vi "Database.Main.vi"() -> ()   [LabVIEW 2016]
uses:
  Database.Main.Data.ctl
  Database.Main.Data.Status.ctl
  Database.Main.Data.Sets.ctl
  Database.Main.Data.Results.ctl
  Sequence/Sequence.Step.Status.ctl
  ProdaNG/Controls/ProdaNG.Identification.ctl
  ProdaNG/Controls/ProdaNG.ProcessResult.ctl
  ProdaNG/Controls/ProdaNG.ProcessStepResult.ctl
  ProdaNG/Controls/ProdaNG.TestStepResult.ctl
  ProdaNG/Controls/ProdaNG.TestValueResult.ctl
  Database.Main.Data.Variant.ctl
  ProdaNG/Controls/ProdaNG.ProcessStepParam.ctl
  ProdaNG/Controls/ProdaNG.TestStep.ctl
  ProdaNG/Controls/ProdaNG.TestStepParam.ctl
  ProdaNG/Controls/ProdaNG.TestValue.ctl
  Database.Main.Action.ctl
  tools/CitTemplate/citTemplate.errData.ctl
  tools/EventLog/EventLog.EventSource.ctl
  Database.Global.vi
panel:
  out "LastFile":string
  out "error.action":string
  out "error":errorcluster
  out "_loop":i32(ring)=4
  out "action":T1=enum."--- DB ---"
  out "Data":T2 {"Variant"."TS"."TV"."minimum" format="%#.3f"; "Variant"."TS"."TV"."maximum" format="%#.3f"; "Variant"."TS"."TP"."value" format="%#.3f"}
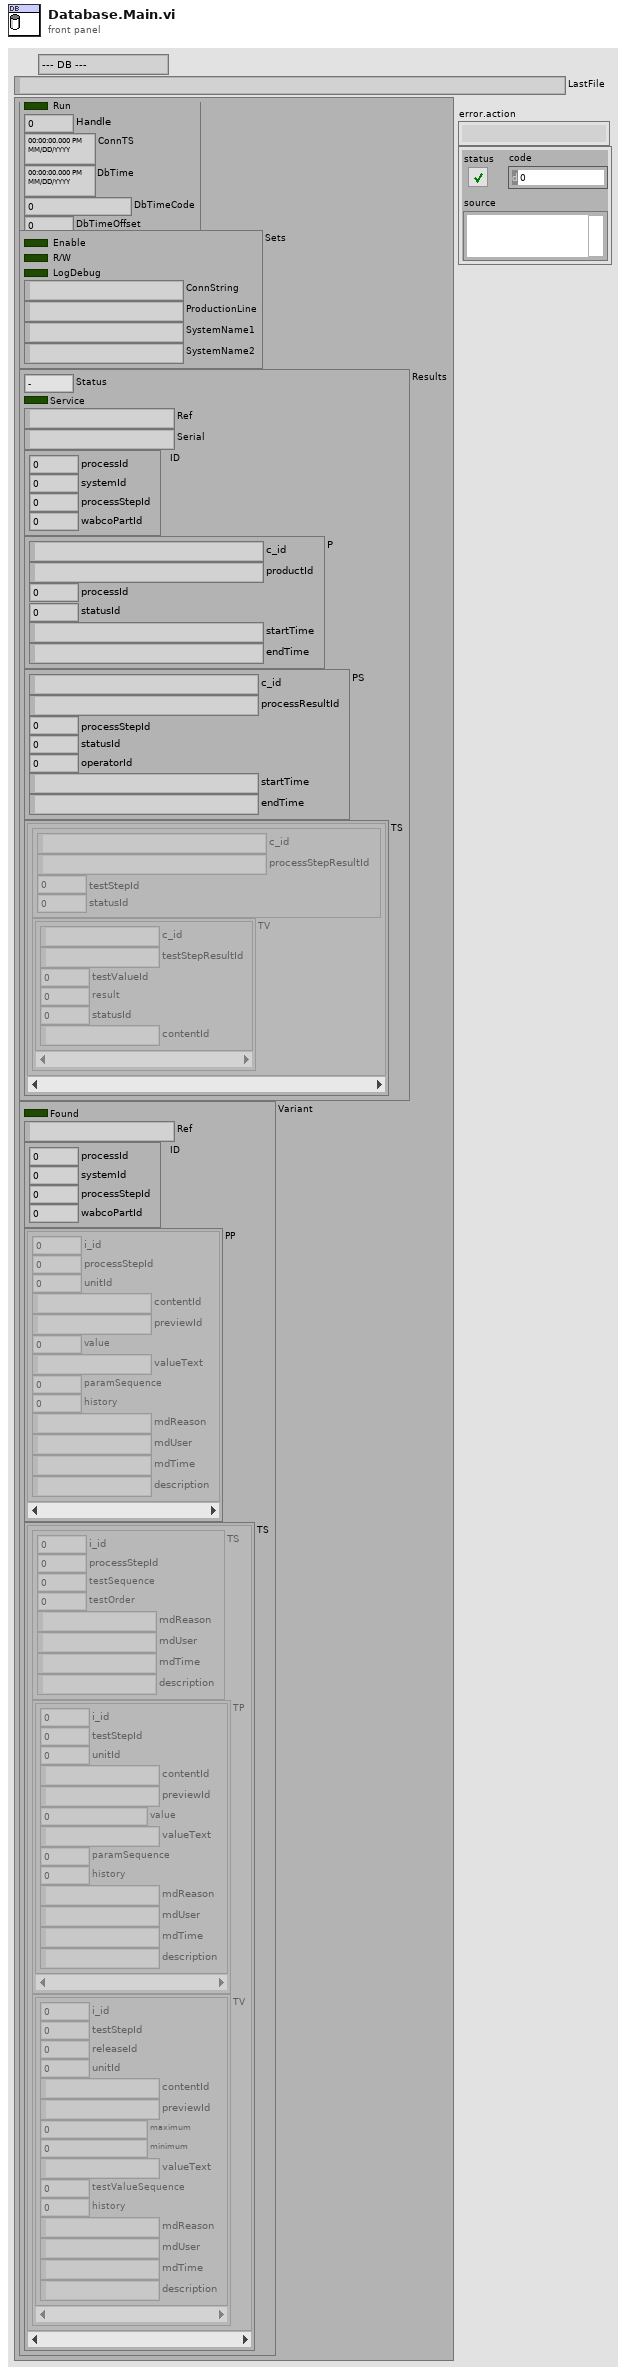
[diagram p1: front panel]
types:
  T1 = typedef "Database.Main.Action.ctl" = enum32{"idle", "constructor", "destructor", "--- DB ---", "Init", "Setup", "Select.Variant", "File.Export"}
  T2 = typedef "Database.Main.Data.ctl" = cluster{"Status":T3, "Sets":T4, "Results":T5, "Variant":T12}
  T3 = typedef "Database.Main.Data.Status.ctl" = cluster{"Run":bool, "Handle":i32, "ConnTS":timestamp, "DbTime":timestamp, "DbTimeCode":dbl, "DbTimeOffset":dbl}
  T4 = typedef "Database.Main.Data.Sets.ctl" = cluster{"Enable":bool, "R/W":bool, "LogDebug":bool, "ConnString":string, "ProductionLine":string, "SystemName1":string, "SystemName2":string}
  T5 = typedef "Database.Main.Data.Results.ctl" = cluster{"Status":T6, "Service":bool, "Ref":string, "Serial":string, "ID":T7, "P":T8, "PS":T9, "TS":cluster{"TS":T10, "TV":T11[]}[]}
  T6 = typedef "Sequence.Step.Status.ctl" = enum16{"-", "Pending", "Running", "Skipped", "Passed", "Failed", "Done", "Error", "Aborted", "Stopped"}
  T7 = typedef "ProdaNG.Identification.ctl" = cluster{"processId":i32, "systemId":i32, "processStepId":i32, "wabcoPartId":i32}
  T8 = typedef "ProdaNG.ProcessResult.ctl" = cluster{"c_id":string, "productId":string, "processId":i32, "statusId":i32, "startTime":string, "endTime":string}
  T9 = typedef "ProdaNG.ProcessStepResult.ctl" = cluster{"c_id":string, "processResultId":string, "processStepId":i32, "statusId":i32, "operatorId":i32, "startTime":string, "endTime":string}
  T10 = typedef "ProdaNG.TestStepResult.ctl" = cluster{"c_id":string, "processStepResultId":string, "testStepId":i32, "statusId":i32}
  T11 = typedef "ProdaNG.TestValueResult.ctl" = cluster{"c_id":string, "testStepResultId":string, "testValueId":i32, "result":dbl, "statusId":i32, "contentId":string}
  T12 = typedef "Database.Main.Data.Variant.ctl" = cluster{"Found":bool, "Ref":string, "ID":T7, "PP":T13[], "TS":cluster{"TS":T14, "TP":T15[], "TV":T16[]}[]}
  T13 = typedef "ProdaNG.ProcessStepParam.ctl" = cluster{"i_id":i32, "processStepId":i32, "unitId":i32, "contentId":string, "previewId":string, "value":dbl, "valueText":string, "paramSequence":i32, "history":i32, "mdReason":string, "mdUser":string, "mdTime":string, "description":string}
  T14 = typedef "ProdaNG.TestStep.ctl" = cluster{"i_id":i32, "processStepId":i32, "testSequence":i32, "testOrder":i32, "mdReason":string, "mdUser":string, "mdTime":string, "description":string}
  T15 = typedef "ProdaNG.TestStepParam.ctl" = cluster{"i_id":i32, "testStepId":i32, "unitId":i32, "contentId":string, "previewId":string, "value":dbl, "valueText":string, "paramSequence":i32, "history":i32, "mdReason":string, "mdUser":string, "mdTime":string, "description":string}
  T16 = typedef "ProdaNG.TestValue.ctl" = cluster{"i_id":i32, "testStepId":i32, "releaseId":i32, "unitId":i32, "contentId":string, "previewId":string, "maximum":dbl, "minimum":dbl, "valueText":string, "testValueSequence":i32, "history":i32, "mdReason":string, "mdUser":string, "mdTime":string, "description":string}
  T17 = typedef "citTemplate.errData.ctl" = cluster{"ts":timestamp, "src":T18, "instance":i32, "action":string, "error":errorcluster, "unconfirmed":bool}
  T18 = typedef "EventLog.EventSource.ctl" = enum16{"All", "Gui", "Ref", "File", "Arch", "Seq", "CPX", "DB", "Laser", "Scan.P", "Scan.O"}
  T19 = typedef "citTemplate.notifierHandle.ctl" = refnum<notifier>
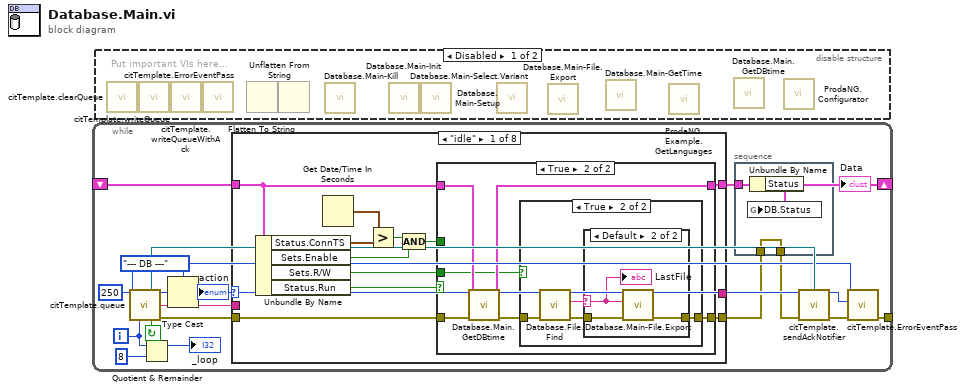
[diagram p0: block diagram]
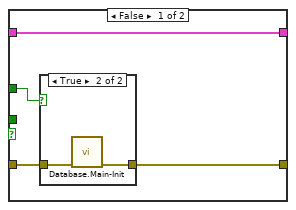
[diagram p3: hidden frame]
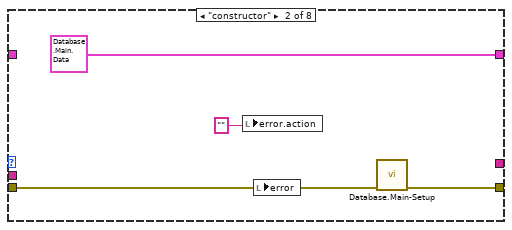
[diagram p7: hidden frame]
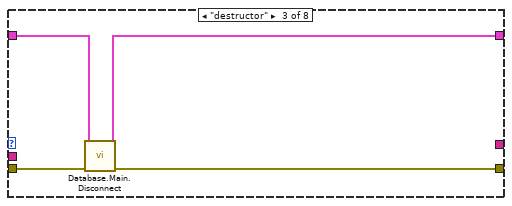
[diagram p8: hidden frame]
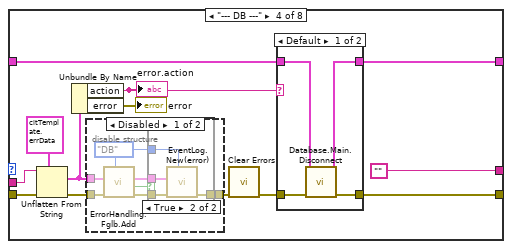
[diagram p9: hidden frame]
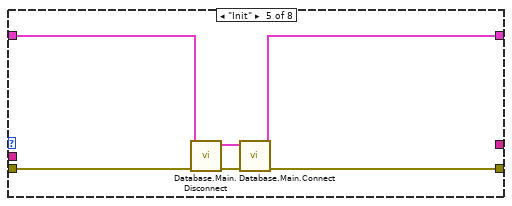
[diagram p13: hidden frame]
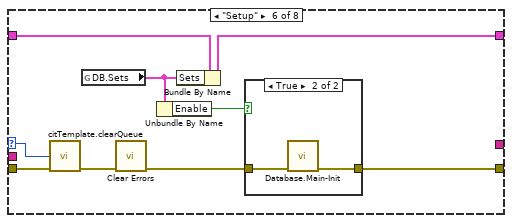
[diagram p14: hidden frame]
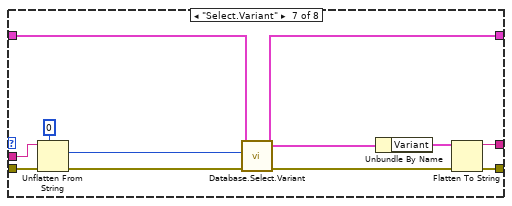
[diagram p16: hidden frame]
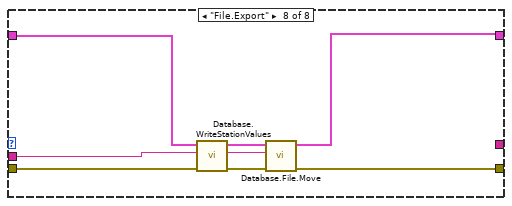
[diagram p17: hidden frame]
diagram:
  n1 = while {
    tunnel: [w11] -> _
    shift-right: [w8] -> _
    shift-left: _ -> [w1]
    i -> [w12]
    stop <- w14 continue-if-true
    w4 = Database.Main.Action."--- DB ---" ("Action")
    n2 = call "citTemplate.queue.vi"("ms timeout (250 ms)"=250, "event enum"=w4, "iteration (-1)"=w12) -> ("notifierHandle out"=w5:T19, "event out"=w17:u32, "(flatten) data out"=w16:string, "continue"=w14:bool, "error out"=w15:errorcluster)  [unwired: 2 in, 6 out]
    n3 = Quotient & Remainder(x=w12, y=8) -> (x-y*floor(x/y)=→"_loop":i32)  [unwired: 1 out]
    n4 = Type Cast(type=w4, x=w17) -> (*(type *) &x=w10:T1)
    "action" <- w10
    n5 = case shown="\"idle\"" w10 {
      selector: w10 -> [_ _ _ _ _ w106 _ _]
      tunnel: w16 -> [_ _ _ w68 _ _ w120 w124]
      tunnel: w15 -> [w29 w54 w59 w74 w94 w107 w121 w128]
      tunnel: [w26 w57 w58 w70 w98 w103 w116 w125] -> w3
      tunnel: [w24 T2 {"Status"={"Run"=FALSE, "Handle"=0, "ConnTS"=timestamp(0 s since 1904-01-01), "DbTime"=timestamp(0 s since 1904-01-01), "DbTimeCode"=0.0, "DbTimeOffset"=0.0}, "Sets"={"Enable"=FALSE, "R/W"=FALSE, "LogDebug"=FALSE, "ConnString"="", "ProductionLine"="", "SystemName1"="", "SystemName2"=""}, "Results"={"Status"=enum."-", "Service"=FALSE, "Ref"="", "Serial"="", "ID"={"processId"=0, "systemId"=0, "processStepId"=0, "wabcoPartId"=0}, "P"={"c_id"="", "productId"="", "processId"=0, "statusId"=0, "startTime"="", "endTime"=""}, "PS"={"c_id"="", "processResultId"="", "processStepId"=0, "statusId"=0, "operatorId"=0, "startTime"="", "endTime"=""}, "TS"=[]}, "Variant"={"Found"=FALSE, "Ref"="", "ID"={"processId"=0, "systemId"=0, "processStepId"=0, "wabcoPartId"=0}, "PP"=[], "TS"=[]}} ("Data") w60 w71 w97 w101 w111 w127] -> w8
      tunnel: w1 -> [w25 _ w61 w72 w93 w102 w118 w126]
      tunnel: [_ _ _ "" _ _ w115 _] -> w6
      frame "idle" {
        n6 = Unbundle By Name(w25) -> ("Status.ConnTS"=w30:timestamp, "Sets.Enable"=w22:bool, "Sets.R/W"=w21:bool, "Status.Run"=w27:bool)
        n7 = Get Date/Time In Seconds() -> (seconds since 1Jan1904=w31:timestamp)
        n8 = Greater?(x=w31, y=w30) -> (0:w28:bool)
        n9 = Compound Arithmetic op=AND(w28, w22) -> (w23:bool)
        n10 = case shown="True" w27 {
          tunnel: w29 -> [w35 w42]
          tunnel: w23 -> [w34 _]
          tunnel: [w33 w40] -> w26
          tunnel: w25 -> [w32 w44]
          tunnel: [w32 w43] -> w24
          tunnel: w21 -> [_ w39]
          frame False {
            n11 = case shown="True" w34 {
              tunnel: w35 -> [w36 w38]
              tunnel: [w36 w37] -> w33
              frame False {
              }
              frame True {
                n12 = call "Database.Main-Init.vi"("error in"=w38) -> ("error out"=w37:errorcluster)  [unwired: 10 in]
              }
            }
          }
          frame True {
            n13 = call "Database.Main.GetDBtime.vi"("error in (no error)"=w42, "Data in"=w44) -> ("error out"=w41:errorcluster, "Data out"=w43:T2)  [unwired: 8 in]
            n14 = case shown="True" w39 {
              tunnel: w41 -> [w45 w49]
              tunnel: [w45 w48] -> w40
              frame False {
              }
              frame True {
                n15 = call "Database.File.Find.vi"("error in (no error)"=w49) -> ("error out"=w47:errorcluster, "FileName"=w46:string)  [unwired: 9 in]
                n16 = case shown="Default" w46 {
                  selector: w46 -> [_ w51]
                  tunnel: w47 -> [w50 w53]
                  tunnel: [w50 w52] -> w48
                  frame "" {
                  }
                  frame Default {
                    n17 = call "Database.Main-File.Export.vi"("error in"=w53, "FileName"=w51) -> ("error out"=w52:errorcluster)  [unwired: 9 in]
                    "LastFile" <- w51
                  }
                }
              }
            }
          }
        }
      }
      frame "constructor" {
        n18 = local write "error.action"("" ("error.action")) -> ()
        n19 = local write "error"(w54) -> ()
        n20 = call "Database.Main-Setup.vi"("error in"=w54) -> ("error out"=w57:errorcluster)  [unwired: 10 in]
      }
      frame "destructor" {
        n21 = call "Database.Main.Disconnect.vi"("error in (no error)"=w59, "Data in"=w61) -> ("error out"=w58:errorcluster, "Data out"=w60:T2)  [unwired: 8 in]
      }
      frame "--- DB ---" {
        n22 = Unflatten From String(type=T17 {"ts"=timestamp(0 s since 1904-01-01), "src"=enum."All", "instance"=0, "action"="", "error"={"status"=FALSE, "code"=0, "source"=""}, "unconfirmed"=FALSE} ("ErrData"), binary string=w68, error in (no error)=w74) -> (value=w63:T17, error out=w66:errorcluster)  [unwired: 3 out]
        n23 = Unbundle By Name(w63) -> ("action"=w62:string, "error"=→"error":errorcluster)
        "error.action" <- w62
        n24 = disable-structure shown="Disabled" {
          disable-tunnel: w66 -> [w78 w86]
          disable-tunnel: [w76 w86] -> w65
          disable-tunnel: w63 -> [w75 _]
          frame Disabled {
            w77 = EventLog.EventSource."DB" ("Event source")
            n25 = call "ErrorHandling.Fglb.Add.vi"("Event source"=w77, "error in (no error)"=w78, "Error in"=w75) -> ("error out"=w80:errorcluster, "changed?"=w79:bool)  [unwired: 7 in]
            n26 = case shown="True" w79 {
              tunnel: [w81 w85] -> w76
              tunnel: w75 -> [_ w84]
              tunnel: w80 -> [w81 w83]
              tunnel: w77 -> [_ w82]
              frame False {
              }
              frame True {
                n27 = call "EventLog.New(error).vi"("Source (All)"=w82, "error in"=w83, "ErrData"=w84) -> ("error out"=w85:errorcluster)  [unwired: 8 in]
              }
            }
          }
          frame Enabled {
          }
        }
        n28 = call <vilib>:"Clear Errors.vi"("error in (no error)"=w65) -> ("error out"=w69:errorcluster)  [unwired: 5 in, 1 out]
        n29 = case shown="Default" w62 {
          tunnel: w72 -> [w90 w91]
          tunnel: [w89 w91] -> w71
          tunnel: [w88 w92] -> w70
          tunnel: w69 -> [w87 w92]
          frame Default {
            n30 = call "Database.Main.Disconnect.vi"("error in (no error)"=w87, "Data in"=w90) -> ("error out"=w88:errorcluster, "Data out"=w89:T2)  [unwired: 8 in]
          }
          frame "Process File" {
          }
        }
      }
      frame "Init" {
        n31 = call "Database.Main.Disconnect.vi"("error in (no error)"=w94, "Data in"=w93) -> ("error out"=w95:errorcluster, "Data out"=w96:T2)  [unwired: 8 in]
        n32 = call "Database.Main.Connect.vi"("error in (no error)"=w95, "Data in"=w96) -> ("error out"=w98:errorcluster, "Data out"=w97:T2)  [unwired: 8 in]
      }
      frame "Setup" {
        n33 = call "citTemplate.clearQueue.vi"("event in"=w106, "error in (no error)"=w107) -> ("error out"=w105:errorcluster)  [unwired: 12 in, 1 out]
        n34 = global read "Database.Global.vi" "DB.Sets"() -> (w100:T4)
        n35 = call <vilib>:"Clear Errors.vi"("error in (no error)"=w105) -> ("error out"=w104:errorcluster)  [unwired: 5 in, 1 out]
        n36 = Unbundle By Name(w100) -> ("Enable"=w99:bool)
        n37 = Bundle By Name(cluster=w102, "Sets"=w100) -> (w101:T2)
        n38 = case shown="True" w99 {
          tunnel: w104 -> [w108 w110]
          tunnel: [w108 w109] -> w103
          frame False {
          }
          frame True {
            n39 = call "Database.Main-Init.vi"("error in"=w110) -> ("error out"=w109:errorcluster)  [unwired: 10 in]
          }
        }
      }
      frame "Select.Variant" {
        n40 = Unflatten From String(type=u64 0, binary string=w120, error in (no error)=w121) -> (value=w113:u64, error out=w119:errorcluster)  [unwired: 3 out]
        n41 = call "Database.Select.Variant.vi"("error in"=w119, "Variant"=w113, "Data in"=w118) -> ("error out"=w117:errorcluster, "Data out"=w111:T2)  [unwired: 7 in]
        n42 = Unbundle By Name(w111) -> ("Variant"=w112:T12)
        n43 = Flatten To String(anything=w112, error in (no error)=w117) -> (data string=w115:string, error out=w116:errorcluster)  [unwired: 2 in, 1 out]
      }
      frame "File.Export" {
        n44 = call "Database.WriteStationValues.vi"("error in"=w128, "FileName"=w124, "Data in"=w126) -> ("error out"=w123:errorcluster, "Data out"=w122:T2)  [unwired: 7 in]
        n45 = call "Database.File.Move.vi"("error in (no error)"=w123, "FileName"=w124, "Data in"=w122) -> ("error out"=w125:errorcluster, "Data out"=w127:T2)  [unwired: 7 in]
      }
    }
    "Data" <- w8
    n46 = stacked-sequence {
      tunnel: w8 -> [w20]
      tunnel: [w18] -> w2
      tunnel: w3 -> [w18]
      frame #0 {
        n47 = Unbundle By Name(w20) -> ("Status"=w19:T3)
        n48 = global write "Database.Global.vi" "DB.Status"(w19) -> ()
      }
    }
    n49 = call "citTemplate.sendAckNotifier.vi"("notification data"=w6, "notifierHandle in"=w5, "error in"=w2) -> ()  [unwired: 13 in]
    n50 = call "citTemplate.ErrorEventPass.vi"("error in"=w2, "action of error"=w10, "event in"=w4) -> ("error out"=w11:errorcluster)  [unwired: 2 in, 6 out]
  }
  n51 = disable-structure shown="Disabled" {
    frame Disabled {
      # "Put important VIs here..."
      n52 = call "citTemplate.clearQueue.vi"() -> ()  [unwired: 14 in, 2 out]
      n53 = call "citTemplate.writeQueue.vi"() -> ()  [unwired: 15 in, 1 out]
      n54 = call "citTemplate.writeQueueWithAck.vi"() -> ()  [unwired: 13 in, 3 out]
      n55 = call "citTemplate.ErrorEventPass.vi"() -> ()  [unwired: 11 in, 1 out]
      n56 = Flatten To String() -> ()  [unwired: 4 in, 3 out]
      n57 = Unflatten From String() -> ()  [unwired: 5 in, 3 out]
      n58 = call "Database.Main-Kill.vi"() -> ()  [unwired: 11 in, 1 out]
      n59 = call "Database.Main-Init.vi"() -> ()  [unwired: 11 in, 1 out]
      n60 = call "Database.Main-Setup.vi"() -> ()  [unwired: 11 in, 1 out]
      n61 = call "Database.Main-Select.Variant.vi"() -> ()  [unwired: 10 in, 2 out]
      n62 = call "Database.Main-File.Export.vi"() -> ()  [unwired: 11 in, 1 out]
      n63 = call "Database.Main-GetTime.vi"() -> ()  [unwired: 1 in, 1 out]
      n64 = call "ProdaNG.Example.GetLanguages.vi"() -> ()  [unwired: 12 in]
      n65 = call "Database.Main.GetDBtime.vi"() -> ()  [unwired: 10 in, 2 out]
      n66 = call "ProdaNG.Configurator.vi"() -> ()  [unwired: 12 in]
    }
    frame Enabled {
    }
  }
